vi "GOMDBTS2048 get Trigger Internal Levels.vi"(8 "error in (no error)":errorcluster, 11 "handle":i32) -> (0 "error out":errorcluster, 1 "function return":i32, 2 "maxLevel":dbl, 3 "triggerLevel":dbl)   [LabVIEW 2015, in "GOMDBTS2048.lvlib"]
doc: "GOBTS2048DLL int __stdcall GOMDBTS2048_getTriggerLevel(int handle, int* value);"
uses:
  GOMDBTS2048.lvlib
  runtime/GOMDBTS2048.dll
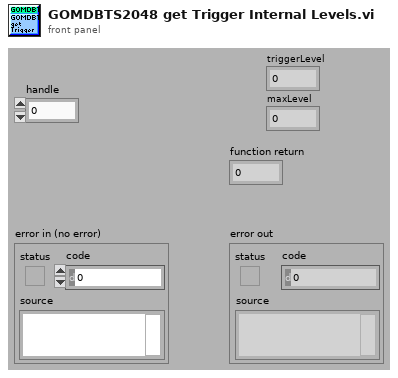
[diagram p1: front panel]
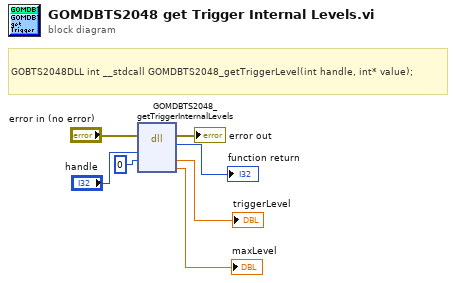
[diagram p0: block diagram]
diagram:
  # "GOBTS2048DLL int __stdcall GOMDBTS2048_getTriggerLevel(int handle, int* value);"
  n1 = dll-call lib="C:/Users/rkoch/Documents/GO_Library/runtime/GOMDBTS2048.*" fn="GOMDBTS2048_getTriggerInternalLevels"(error in="error in (no error)", "handle"="handle", "triggerLevel"=0 ("value")) -> (error out=→"error out":errorcluster, "return type"=→"function return":i32, "triggerLevel"=→"triggerLevel":dbl, "maxLevel"=→"maxLevel":dbl)  [unwired: 4 in, 1 out]
